vi "ATF-Pump-Drive_messsage_A.vi"(10 "Numeric":i32=17, 11 "Switching Freq.":dbl) -> (3 "String":string)   [LabVIEW 2022 SP3]
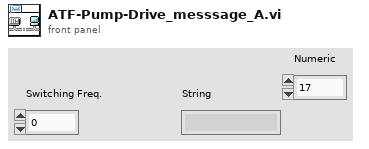
[diagram p1: front panel]
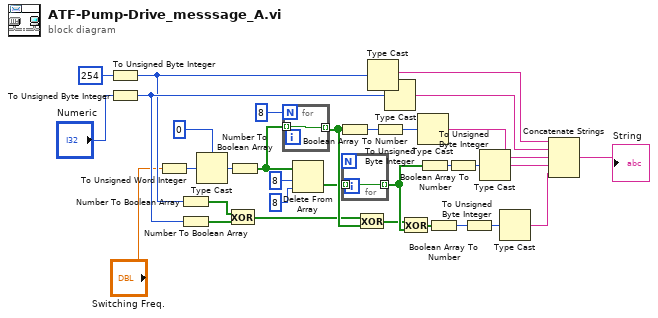
[diagram p0: block diagram]
diagram:
  n1 = To Unsigned Byte Integer(number=254) -> (unsigned 8bit integer=w22:u8)
  n2 = To Unsigned Byte Integer(number="Numeric") -> (unsigned 8bit integer=w23:u8)
  n3 = To Unsigned Word Integer(number="Switching Freq.") -> (unsigned 16bit integer=w24:u16)
  n4 = Number To Boolean Array(number=w22) -> (Boolean array=w20:bool[])
  n5 = Number To Boolean Array(number=w23) -> (Boolean array=w21:bool[])
  n6 = Type Cast(type=i16 0, x=w24) -> (*(type *) &x=w7:i16)
  n7 = Exclusive Or(1:w21, 2:w20) -> (0:w29:bool[])
  n8 = Number To Boolean Array(number=w7) -> (Boolean array=w16:bool[])
  n9 = for {
    N: 8 -> [_]
    tunnel: w16 -> [w33] mode=indexing
    tunnel: [w33] -> w31 mode=indexing
  }
  n10 = Delete From Array(array=w16, length=8, index=8) -> (deleted portion=w13:bool[])  [unwired: 1 out]
  n11 = Boolean Array To Number(Boolean array=w31) -> (number=w11:u32)
  n12 = for {
    tunnel: w13 -> [w34] mode=indexing
    tunnel: [w34] -> w32 mode=indexing
  }
  n13 = Exclusive Or(1:w31, 2:w29) -> (0:w28:bool[])
  n14 = Type Cast(x=w22) -> (*(type *) &x=w4:string)  [unwired: 1 in]
  n15 = To Unsigned Byte Integer(number=w11) -> (unsigned 8bit integer=w10:u8)
  n16 = Type Cast(x=w23) -> (*(type *) &x=w5:string)  [unwired: 1 in]
  n17 = Exclusive Or(1:w32, 2:w28) -> (0:w27:bool[])
  n18 = Type Cast(x=w10) -> (*(type *) &x=w12:string)  [unwired: 1 in]
  n19 = Boolean Array To Number(Boolean array=w32) -> (number=w18:u32)
  n20 = Boolean Array To Number(Boolean array=w27) -> (number=w26:u32)
  n21 = To Unsigned Byte Integer(number=w18) -> (unsigned 8bit integer=w17:u8)
  n22 = To Unsigned Byte Integer(number=w26) -> (unsigned 8bit integer=w25:u8)
  n23 = Type Cast(x=w17) -> (*(type *) &x=w19:string)  [unwired: 1 in]
  n24 = Type Cast(x=w25) -> (*(type *) &x=w30:string)  [unwired: 1 in]
  n25 = Concatenate Strings(w4, w5, w12, w19, w30) -> (→"String":string)
